vi "FF.vi"(2 "Q_prev":dbl, 3 "Enable":bool, 5 "D":dbl) -> (1 "Q":dbl)   [LabVIEW 2020]
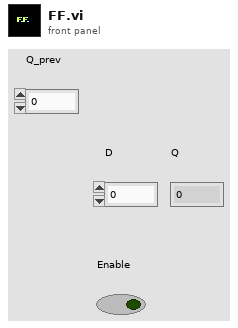
[diagram p1: front panel]
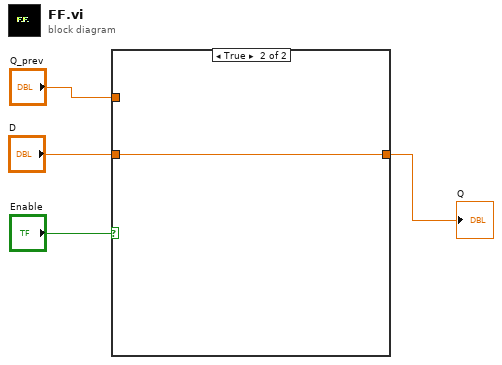
[diagram p0: block diagram]
diagram:
  n1 = case shown="False" "Enable" {
    tunnel: "D" -> [_ w6]
    tunnel: [w5 w6] -> w2
    tunnel: "Q_prev" -> [w5 _]
    frame False {
    }
    frame True {
    }
  }
  "Q" <- w2
